vi "Main.vi"() -> ()   [LabVIEW 2016]
panel:
  out "数值 2":dbl
  in  "上取整(F)":bool
  in  "停止":bool
  out "波形图表":i64(graph)
  out "数值":dbl
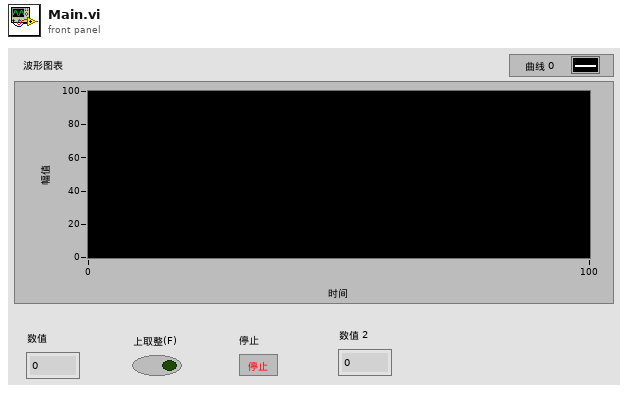
[diagram p1: front panel]
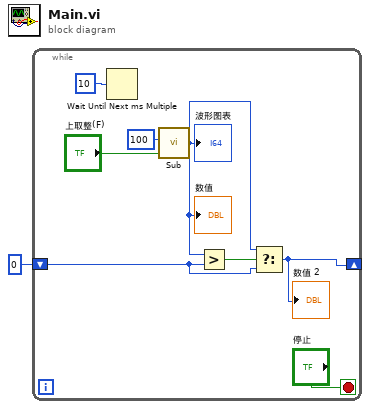
[diagram p0: block diagram]
diagram:
  n1 = while {
    shift-right: [w3] -> _
    shift-left: 0 -> [w4]
    stop <- "停止" stop-if-true
    n2 = Wait Until Next ms Multiple(millisecond multiple=u32 10 ("毫秒倍数")) -> ()  [unwired: 1 out]
    n3 = call "Sub.vi"("上取整(F)"="上取整(F)", "最大值"=i64 100) -> ("随机生成的整数"=w5:i64)  [unwired: 3 in]
    "数值" <- w5
    "波形图表" <- w5
    n4 = Greater?(x=w5, y=w4) -> (0:w6:bool)
    n5 = Select(t=w5, s=w6, f=w4) -> (s? t:f=w3:i64)
    "数值 2" <- w3
  }
